vi "UI_guessLetter_enableOK.vi"(8 "Accept":refnum<vi>, 10 "charDiscarded?":bool, 11 "Letter":refnum<vi>) -> ()   [LabVIEW 2020]
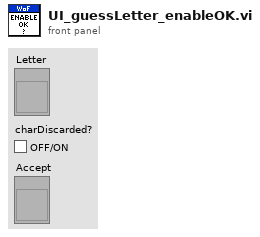
[diagram p1: front panel]
types:
  T1 = enum8{"Enabled", "Disabled", "Disabled and Grayed Out"}
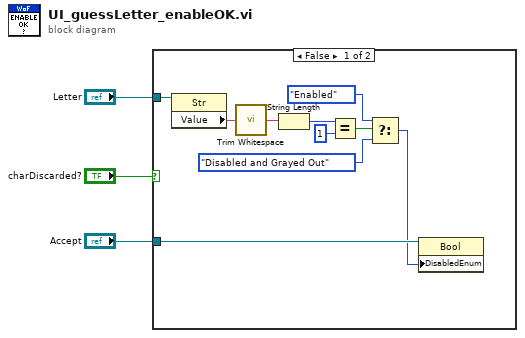
[diagram p0: block diagram]
diagram:
  n1 = case shown="False" "charDiscarded?" {
    tunnel: "Letter" -> [w13 _]
    tunnel: "Accept" -> [w8 _]
    frame False {
      n2 = property class="Str"(reference=w13) -> ("Value"=w12:string)  [unwired: 1 in, 2 out]
      n3 = call <vilib>:"Trim Whitespace.vi"("string"=w12) -> ("trimmed string"=w11:string)  [unwired: 1 in]
      n4 = String Length(string=w11) -> (length=w10:i32)
      n5 = Equal?(x=w10, y=1) -> (x = y?=w7:bool)
      n6 = Select(t=T1."Enabled" ("Disabled"), s=w7, f=T1."Disabled and Grayed Out" ("Disabled")) -> (s? t:f=w4:T1)
      n7 = property class="Bool"(reference=w8, "DisabledEnum"=w4) -> ()  [unwired: 1 in, 2 out]
    }
    frame True {
    }
  }
